vi "Array Fraction.vi"(6 "Direction (from start)":enum16{"from start", "from end"}(ring), 8 "Error In":errorcluster, 9 "fraction [0, 1]":dbl min=0.0 max=1.0, 10 "Method (Length Based)":enum16{"Value Based", "Length Based"}(ring)=enum."Length Based", 11 "Array":dbl[](array[numeric])) -> (0 "Error Out":errorcluster, 3 "Array out":dbl[](array[numeric]))   [LabVIEW 2021, in "Arrays.lvlib"]
doc: "Returns part of the input <B>Array</B> ([Ai]), according the the following rules:\n\n- if <B>Method</B> is <B>Value Based</B>, returns (possibly non-consecutive) array values Ai such that:\n Ai - Min <= (Max-Min)*fraction (<B>from start</B>) \n or Ai - Min => (Max - Min)*fraction (<B>from end</B>)\n\n- if if <B>Method</B> is <B>Length Based</B> (default), returns N*fraction elements of the array (where N is the array size) starting from the end or the beginning, depending on the <B>Direction</B> parameter (default: <B>from start</B>)"
uses:
  Arrays.lvlib
panel:
  out "fraction out":dbl
  # "see the AlliGator License on the block diagram (Ctrl+E or Window:Show Block Diagram)"
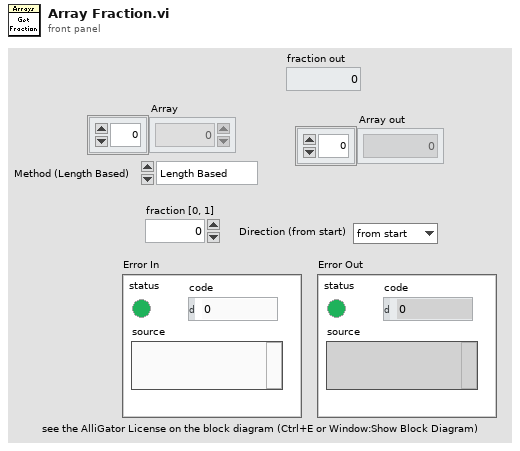
[diagram p1: front panel]
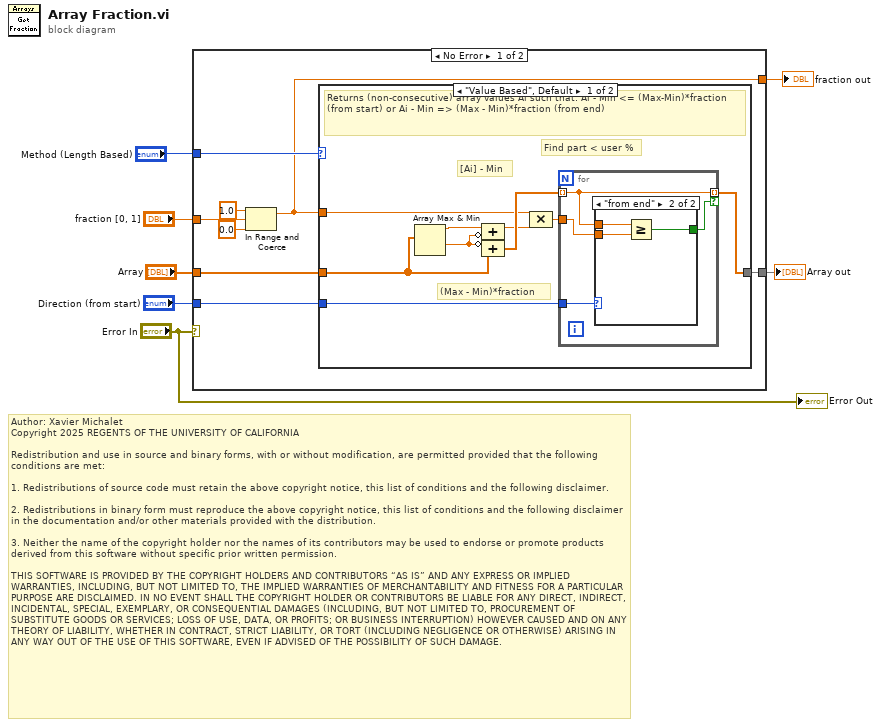
[diagram p0: block diagram]
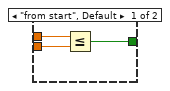
[diagram p2: hidden frame]
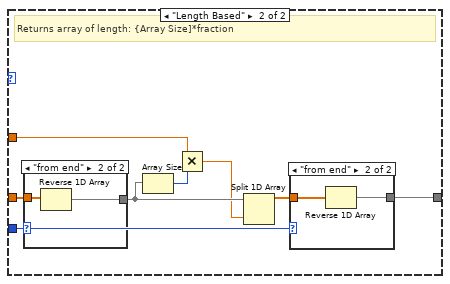
[diagram p3: hidden frame]
diagram:
  # "Author: Xavier Michalet\nCopyright 2025 REGENTS OF THE UNIVERSITY OF CALIFORNIA\n\nRedistribution and use in source and binary forms, with or without modification, are permitted provided that the following conditions are met:\n\n1. Redistributions of source code must retain the above copyright notice, this list of conditions and the following disclaimer.\n\n2. Redistributions in binary form must reproduce the above copyright notice, this list of conditions and the following disclaimer in the documentation and/or other materials provided with the distribution.\n\n3. Neither the name of the copyright holder nor the names of its contributors may be used to endorse or promote products derived from this software without specific prior written permission.\n\nTHIS SOFTWARE IS PROVIDED BY THE COPYRIGHT HOLDERS AND CONTRIBUTORS “AS IS” AND ANY EXPRESS OR IMPLIED WARRANTIES, INCLUDING, BUT NOT LIMITED TO, THE IMPLIED WARRANTIES OF MERCHANTABILITY AND FITNESS FOR A PARTICULAR PURPOSE ARE DISCLAIMED. IN NO EVENT SHALL THE COPYRIGHT HOLDER OR CONTRIBUTORS BE LIABLE FOR ANY DIRECT, INDIRECT, INCIDENTAL, SPECIAL, EXEMPLARY, OR CONSEQUENTIAL DAMAGES (INCLUDING, BUT NOT LIMITED TO, PROCUREMENT OF SUBSTITUTE GOODS OR SERVICES; LOSS OF USE, DATA, OR PROFITS; OR BUSINESS INTERRUPTION) HOWEVER CAUSED AND ON ANY THEORY OF LIABILITY, WHETHER IN CONTRACT, STRICT LIABILITY, OR TORT (INCLUDING NEGLIGENCE OR OTHERWISE) ARISING IN ANY WAY OUT OF THE USE OF THIS SOFTWARE, EVEN IF ADVISED OF THE POSSIBILITY OF SUCH DAMAGE."
  n1 = case shown="No Error" "Error In" {
    tunnel: "Array" -> [w15 w50]
    tunnel: [w14 w50] -> w6
    tunnel: "fraction [0, 1]" -> [w13 w49]
    tunnel: "Direction (from start)" -> [w12 _]
    tunnel: "Method (Length Based)" -> [w11 _]
    tunnel: [w8 w49] -> w1
    frame No Error {
      n2 = In Range and Coerce(upper limit=1.0, x=w13, lower limit=0.0) -> (coerced(x)=w8:dbl)  [unwired: 1 out]
      n3 = case shown="\"Value Based\", Default" w11 {
        tunnel: w15 -> [w24 w42]
        tunnel: [w20 w36] -> w14
        tunnel: w8 -> [w18 w41]
        tunnel: w12 -> [w16 w35]
        frame "Value Based", Default {
          # "(Max - Min)*fraction"
          # "[Ai] - Min"
          # "Find part < user %"
          # "Returns (non-consecutive) array values Ai such that: Ai - Min <= (Max-Min)*fraction (from start) or Ai - Min => (Max - Min)*fraction (from end)"
          n4 = Array Max & Min(array=w24) -> (max value=w22:dbl, min value=w21:dbl)  [unwired: 2 out]
          n5 = Compound Arithmetic op=ADD(w22, invert w21) -> (w19:dbl)
          n6 = Compound Arithmetic op=ADD(invert w21, w24) -> (w23:dbl[])
          n7 = Compound Arithmetic op=MULTIPLY(w18, w19) -> (w17:dbl)
          n8 = for {
            tunnel: w23 -> [w28] mode=indexing
            tunnel: [w28] -> w20 mode=indexing if=w27
            tunnel: w17 -> [w26]
            tunnel: w16 -> [w25]
            n9 = case shown="\"from end\"" w25 {
              tunnel: w28 -> [w31 w34]
              tunnel: [w30 w33] -> w27
              tunnel: w26 -> [w29 w32]
              frame "from start", Default {
                n10 = Less Or Equal?(x=w31, y=w29) -> (x <= y?=w30:bool)
              }
              frame "from end" {
                n11 = Greater Or Equal?(x=w34, y=w32) -> (x >= y?=w33:bool)
              }
            }
          }
        }
        frame "Length Based" {
          # "Returns array of length: {Array Size]*fraction"
          n12 = case shown="\"from end\"" w35 {
            tunnel: w42 -> [w46 w48]
            tunnel: [w46 w47] -> w39
            frame "from start", Default {
            }
            frame "from end" {
              n13 = Reverse 1D Array(array=w48) -> (reversed array=w47:dbl[])
            }
          }
          n14 = Array Size(array=w39) -> (size(s)=w40:i32)
          n15 = Multiply(x=w41, y=w40) -> (x*y=w38:dbl)
          n16 = Split 1D Array(array=w39, index=w38) -> (first subarray=w37:dbl[])  [unwired: 1 out]
          n17 = case shown="\"from end\"" w35 {
            tunnel: w37 -> [w43 w45]
            tunnel: [w43 w44] -> w36
            frame "from start", Default {
            }
            frame "from end" {
              n18 = Reverse 1D Array(array=w45) -> (reversed array=w44:dbl[])
            }
          }
        }
      }
    }
    frame Error {
    }
  }
  "Array out" <- w6
  "fraction out" <- w1
  "Error Out" <- "Error In"
